vi "Oscilloscope.vi"() -> ()   [LabVIEW 2018]
uses:
  <instrlib>/LeCroy Wave Series/Public/Data/Read Single Waveform.vi
  <instrlib>/LeCroy Wave Series/LeCroy Wave Series.lvlib
panel:
  in  "Save Files in Directory":string="D:\\Automation\\Data"
  out "Saved filename":string
  in  "VISA resource name":refnum<visa-resource-name>
  in  "Reset Scope?":bool
  in  "Perform Auto Setup?":bool
  in  "Source (0: Channel 1)":u16(ring) items=["Channel 1", "Channel 2", "Channel 3", "Channel 4", "Memory 1", "Memory 2", "Memory 3", "Memory 4", "Function 1", "Function 2", "Function 3", "Function 4", "Function 5", "Function 6", "Function 7", "Function 8"]
  in  "Timeout (10000 ms)":u32=10000
  out "Waveform Data":waveform(dbl)(graph)
  in  "stop":bool
  out ".not. x?":bool
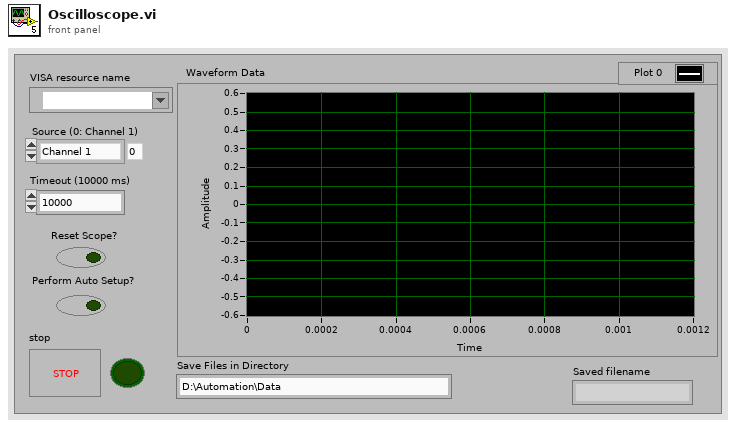
[diagram p1: front panel]
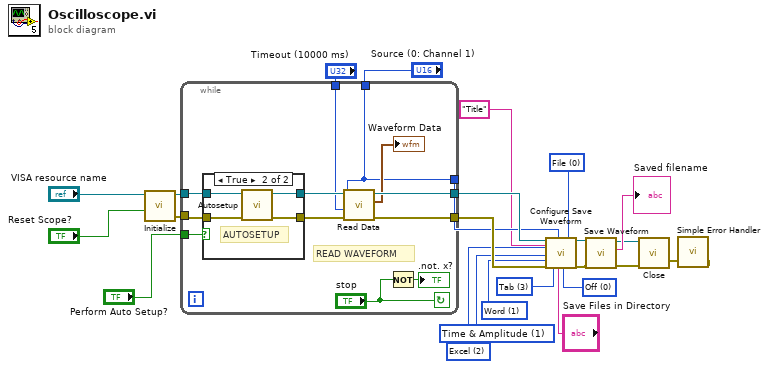
[diagram p0: block diagram]
diagram:
  w7 = u16 3 items=["Comma", "Space", "Semicolon", "Tab"] ("Delimiter (  0:Comma)")
  w8 = u16 0 items=["Off", "Wrap", "Fill"] ("Auto Save (0:Off")
  w9 = u16 1 items=["Byte", "Word", "Auto"] ("BinarySubFormat (1: Word)")
  w11 = u16 1 items=["Amplitude Only", "Time & Amplitude", "With Header"] ("SubFormat (1: Time & Amplitude)")
  w12 = u16 2 items=["Binary", "ASCII", "Excel", "MATLAB", "MathCad", "WaveML"] ("Format (0: Binary)")
  w13 = u16 0 items=["File", "M1", "M2", "M3", "M4"] ("Destination (0:File)")
  n1 = call <instrlib>:"Initialize.vi"("Reset? (T: Yes)"="Reset Scope?", "VISA resource name"="VISA resource name") -> ("error out"=w21:errorcluster, "VISA resource name out"=w22:refnum<visa-resource-name>)  [unwired: 8 in]
  n2 = while {
    tunnel: [w34] -> w15
    tunnel: [w33] -> w16
    tunnel: "Perform Auto Setup?" -> [w32]
    tunnel: "Source (0: Channel 1)" -> [w25]
    tunnel: w21 -> [w31]
    tunnel: w22 -> [w30]
    tunnel: "Timeout (10000 ms)" -> [w29]
    tunnel: [w25] -> w14
    stop <- "stop" continue-if-true
    # "READ WAVEFORM"
    n3 = case shown="True" w32 {
      tunnel: w31 -> [w37 w42]
      tunnel: w30 -> [w38 w41]
      tunnel: [w38 w40] -> w36
      tunnel: [w37 w39] -> w35
      frame False {
      }
      frame True {
        # "AUTOSETUP"
        n4 = call <instrlib>:"Autosetup.vi"("error in (no error)"=w42, "VISA resource name"=w41) -> ("error out"=w39:errorcluster, "VISA resource name out"=w40:refnum<visa-resource-name>)  [unwired: 8 in]
      }
    }
    n5 = call-poly <instrlib>:"Read Data.vi"("error in (no error)"=w35, "Timeout (10000 ms)"=w29, "Source (0: Channel 1)"=w25, "VISA resource name"=w36) -> ("error out"=w34:errorcluster, "Waveform Data"=→"Waveform Data":waveform(dbl), "VISA resource name out"=w33:refnum<visa-resource-name>)  [unwired: 5 in]
    n6 = Not(x="stop") -> (.not. x?=→".not. x?":bool)
  }
  n7 = call <instrlib>:"Configure Save Waveform.vi"("VISA resource name"=w16, "Trace Title (Title)"="Title", "Format (0: Binary)"=w12, "SubFormat (1: Time & Amplitude)"=w11, "BinarySubFormat (1: Word)"=w9, "error in (no error)"=w15, "Delimiter (  0:Comma)"=w7, "Source (0: Channel 1)"=w14, "Save Files in Directory (D:\\Waveforms)"="Save Files in Directory", "Auto Save (0:Off"=w8, "Destination (0:File)"=w13) -> ("VISA resource name out"=w5:refnum<visa-resource-name>, "error out"=w4:errorcluster)  [unwired: 7 in]
  n8 = call <instrlib>:"Save Waveform.vi"("error in (no error)"=w4, "VISA resource name"=w5) -> ("error out"=w1:errorcluster, "Saved filename"=→"Saved filename":string, "VISA resource name out"=w2:refnum<visa-resource-name>)  [unwired: 7 in]
  n9 = call <instrlib>:"Close.vi"("error in (no error)"=w1, "VISA resource name"=w2) -> ("error out"=w24:errorcluster)  [unwired: 9 in]
  n10 = call <vilib>:"Simple Error Handler.vi"("error in (no error)"=w24) -> ()  [unwired: 4 in, 5 out]
